vi "Is Done.vi"(8 "Error In":errorcluster, 11 "Reader In":refnum<class "Abstract.lvclass">) -> (0 "Error Out":errorcluster, 2 "Done":bool, 3 "Reader Out":refnum<class "Abstract.lvclass">)   [LabVIEW 2018, in "Toolkit.lvlib" / "Readers.lvlib" / "Abstract.lvclass"]
doc: "Indicates if there is more template to read."
uses:
  Abstract.lvclass
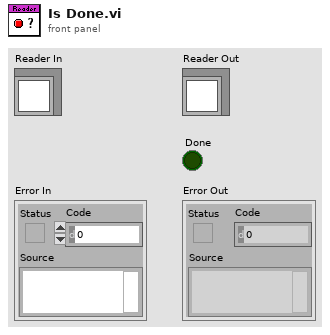
[diagram p1: front panel]
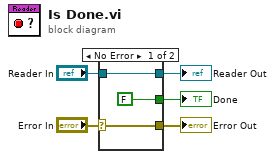
[diagram p0: block diagram]
diagram:
  n1 = case shown="No Error" "Error In" {
    selector: "Error In" -> [w7 w10]
    tunnel: [w7 w10] -> w4
    tunnel: [w8 w9] -> w2
    tunnel: "Reader In" -> [w8 w9]
    tunnel: [FALSE _] -> w1
    frame No Error {
    }
    frame Error {
    }
  }
  "Error Out" <- w4
  "Reader Out" <- w2
  "Done" <- w1
